vi "LeseWegzähler.vi"(8 "error in (no error)":errorcluster caption="Fehler (Eingang, kein Fehler)") -> (0 "error out":errorcluster caption="Fehler (Ausgang)", 2 "Zeit für Service":bool, 3 "value":dbl caption="Wegzähler")   [LabVIEW 2014]
uses:
  <vilib>/Utility/config.llb/Read Key (Double).vi
  <vilib>/Utility/config.llb/NI_LVConfig.lvlib
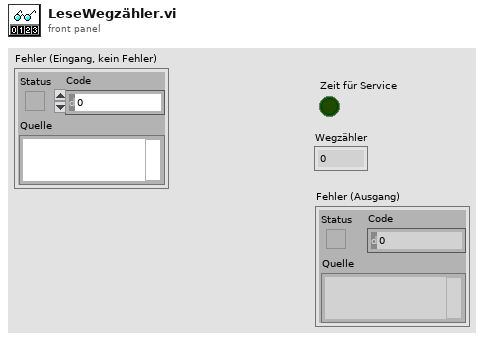
[diagram p1: front panel]
types:
  T1 = typedef "NI_LVConfig.lvlib/Config Data RefNum.ctl" = refnum<k1>
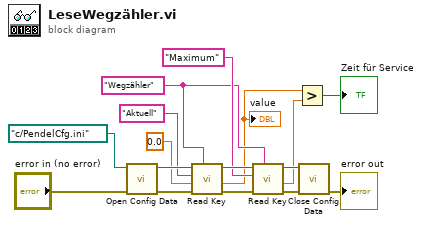
[diagram p0: block diagram]
diagram:
  w3 = "Wegzähler" ("section")
  n1 = call <vilib>:"Open Config Data.vi"("error in (no error)"="error in (no error)", "configuration file path"=path "c:/PendelCfg.ini") -> ("error out"=w14:errorcluster, "refnum"=w15:T1)  [unwired: 7 in, 1 out]
  n2 = call-poly <vilib>:"Read Key.vi"("section"=w3, "error in (no error)"=w14, "default value"=0.0, "key"="Aktuell", "refnum"=w15) -> ("error out"=w13:errorcluster, "value"=w2:dbl, "refnum out"=w12:T1)  [unwired: 3 in, 1 out]
  "value" <- w2
  n3 = call-poly <vilib>:"Read Key.vi"("section"=w3, "error in (no error)"=w13, "key"="Maximum", "refnum"=w12) -> ("error out"=w9:errorcluster, "value"=w7:dbl, "refnum out"=w8:T1)  [unwired: 4 in, 1 out]
  n4 = Greater?(x=w2, y=w7) -> (0:→"Zeit für Service":bool)
  n5 = call <vilib>:"Close Config Data.vi"("error in (no error)"=w9, "refnum"=w8) -> ("error out"=→"error out":errorcluster)  [unwired: 8 in, 1 out]
